vi "Peak Detection Helper.vi"(8 "Error In":errorcluster, 9 "threshold":dbl format="%.2p", 10 "Waveform":waveform(dbl)) -> (0 "Error Out":errorcluster, 2 "Annotations":T1(array[cluster]))   [LabVIEW 2013, in "Diode Characterization.lvlib" / "Diode IV.lvclass"]
doc: "Detects up to 10 peaks in the given waveform that are over the given threshold. Output is in the form of an array of annotations that can be displayed on the graph alongside the input waveform."
uses:
  Diode IV.lvclass
  <vilib>/measure/mamon.llb/Waveform Peak Detection for 1 Chan.vi
  <vilib>/measure/NI_MAPro.lvlib
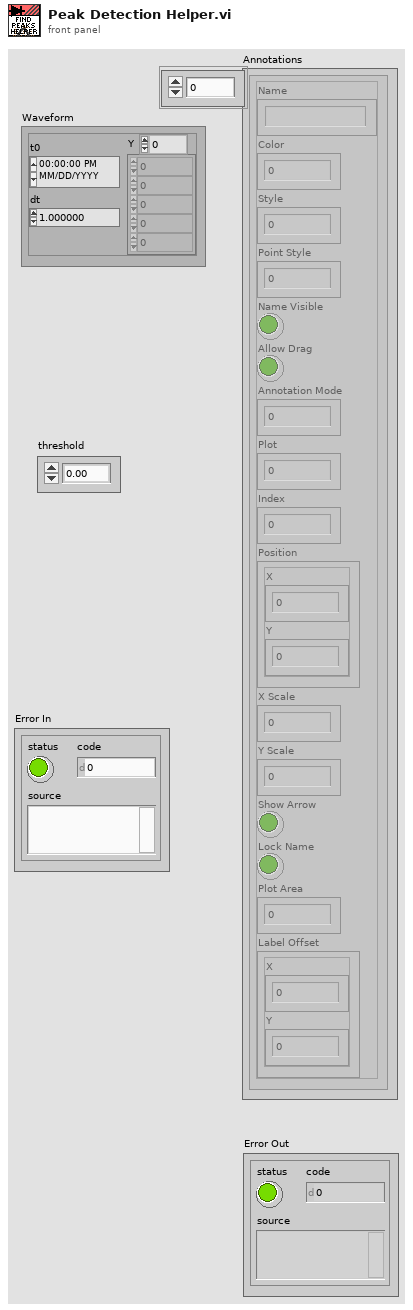
[diagram p1: front panel]
types:
  T1 = cluster{"Name":string, "Color":u32, "Style":u8, "Point Style":u8, "Name Visible":bool, "Allow Drag":bool, "Annotation Mode":u32, "Plot":i32, "Index":i32, "Position":cluster{"X":dbl, "Y":dbl}, "X Scale":u32, "Y Scale":u32, "Show Arrow":bool, "Lock Name":bool, "Plot Area":i32, "Label Offset":cluster{"X":dbl, "Y":dbl}}[]
  T2 = cluster{"Name":string, "Color":u32, "Style":u8, "Point Style":u8, "Name Visible":bool, "Allow Drag":bool, "Annotation Mode":u32, "Plot":i32, "Index":i32, "Position":cluster{"X":dbl, "Y":dbl}, "X Scale":u32, "Y Scale":u32, "Show Arrow":bool, "Lock Name":bool, "Plot Area":i32, "Label Offset":cluster{"X":dbl, "Y":dbl}}
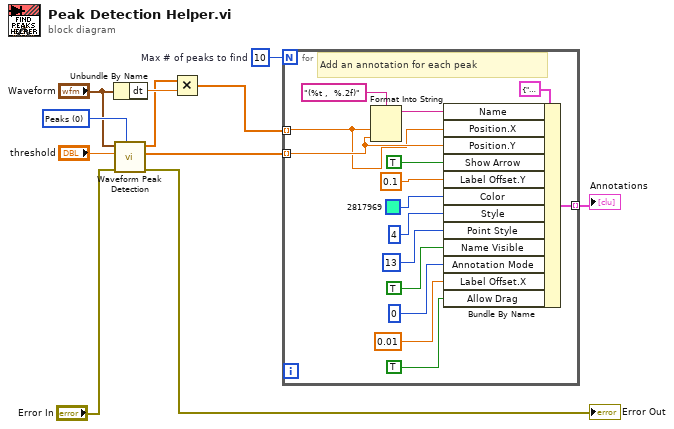
[diagram p0: block diagram]
diagram:
  w4 = 10  # Max # of peaks to find
  w10 = u16 0 items=["Peaks", "Valleys"] ("peaks/valleys")
  n1 = Unbundle By Name("Waveform") -> ("dt"=w7:dbl)
  n2 = call-poly <vilib>:"Waveform Peak Detection.vi"("peaks/valleys"=w10, "error in"="Error In", "threshold"="threshold", "Signal In"="Waveform") -> ("error out"=→"Error Out":errorcluster, "Amplitudes"=w11:dbl[], "Locations"=w6:dbl[])  [unwired: 3 in, 2 out]
  n3 = Multiply(x=w6, y=w7) -> (x*y=w5:dbl[])
  n4 = for {
    N: w4 -> [_]
    tunnel: w5 -> [w12] mode=indexing
    tunnel: w11 -> [w13] mode=indexing
    tunnel: [w25] -> w9 mode=indexing
    # "Add an annotation for each peak"
    n5 = Format Into String(format string="(%t ,  %.2f)", w12, w13) -> (resulting string=w15:string)  [unwired: 2 in, 1 out]
    n6 = Bundle By Name(cluster=T2 {"Name"="", "Color"=0, "Style"=0, "Point Style"=0, "Name Visible"=FALSE, "Allow Drag"=FALSE, "Annotation Mode"=0, "Plot"=0, "Index"=0, "Position"={"X"=0.0, "Y"=0.0}, "X Scale"=0, "Y Scale"=0, "Show Arrow"=FALSE, "Lock Name"=FALSE, "Plot Area"=0, "Label Offset"={"X"=0.0, "Y"=0.0}} ("element"), "Name"=w15, "Position.X"=w12, "Position.Y"=w13, "Show Arrow"=TRUE, "Label Offset.Y"=0.1, "Color"=u32 2817969, "Style"=u8 4, "Point Style"=u8 13, "Name Visible"=TRUE, "Annotation Mode"=u32 0, "Label Offset.X"=0.01, "Allow Drag"=TRUE) -> (w25:T2)
  }
  "Annotations" <- w9
